vi "Test Register Path.vi"() -> ()   [LabVIEW 2021, in "Path Utilities.lvlib"]
doc: "Unit Test for \"Register Path.vi\"."
uses:
  Path Utilities.lvlib
panel:
  out "Cleared Paths":path[](array[path])
  out "Result":bool
  in  "Tests":T1(tab)
  out "Test 1":T2
  out "Test 2":T2
  out "Test 3":T2
  out "Test 4":T2
  out "Test 5":T2
  out "Test 6":T2
  out "Test 7":T2
  out "Test 8":T2
  out "Test 9":T2
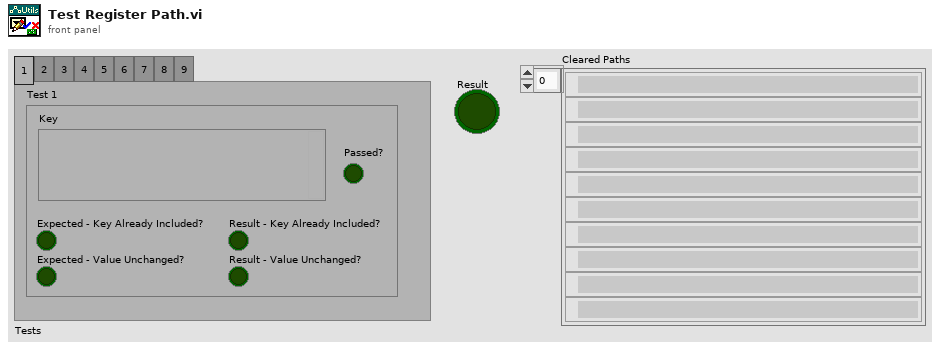
[diagram p1: front panel]
types:
  T1 = enum32{"1", "2", "3", "4", "5", "6", "7", "8", "9"}
  T2 = cluster{"Key":variant, "Result - Key Already Included?":bool, "Result - Value Unchanged?":bool, "Expected - Key Already Included?":bool, "Expected - Value Unchanged?":bool, "Passed?":bool}
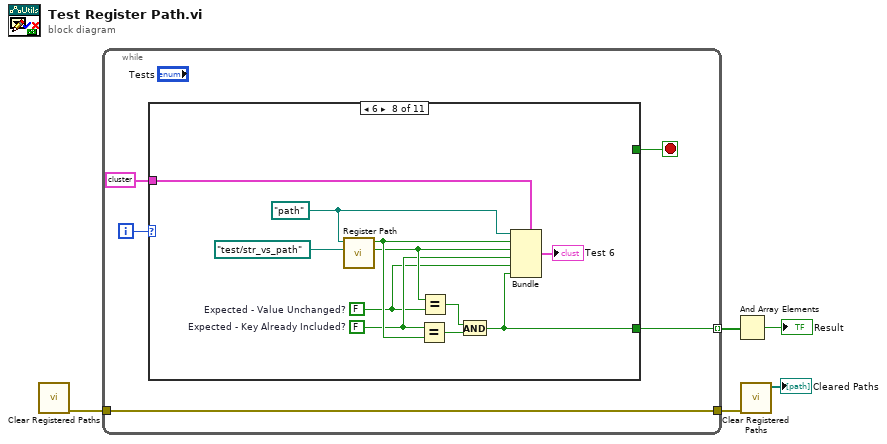
[diagram p0: block diagram]
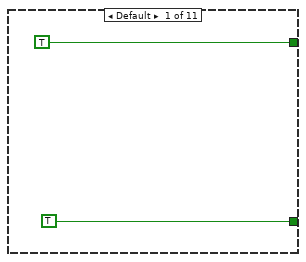
[diagram p2: hidden frame]
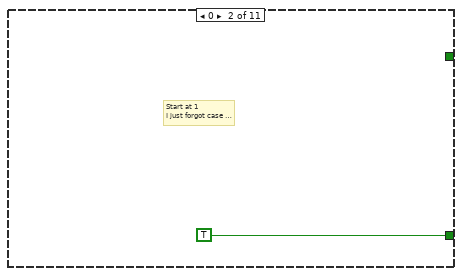
[diagram p3: hidden frame]
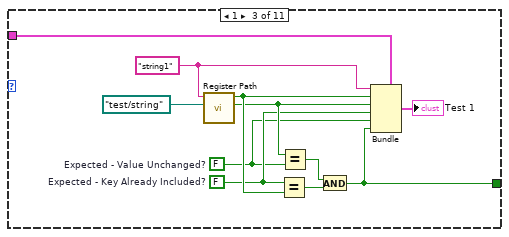
[diagram p4: hidden frame]
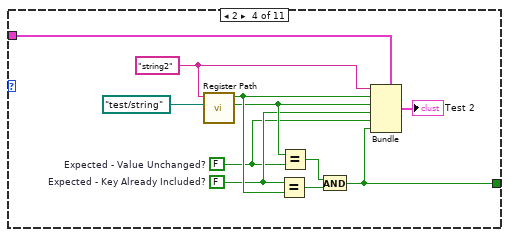
[diagram p5: hidden frame]
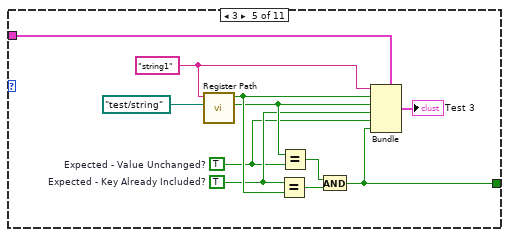
[diagram p6: hidden frame]
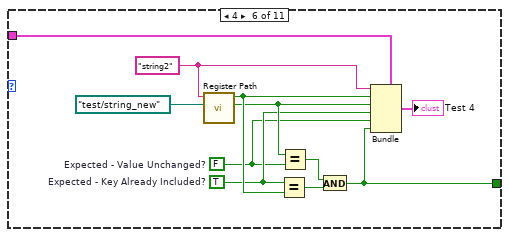
[diagram p7: hidden frame]
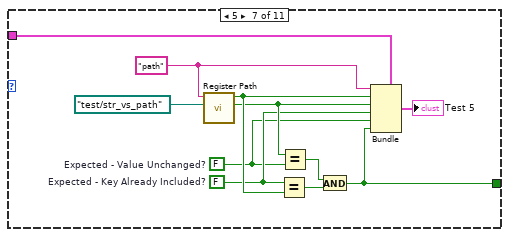
[diagram p8: hidden frame]
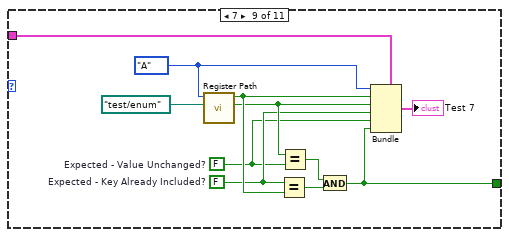
[diagram p9: hidden frame]
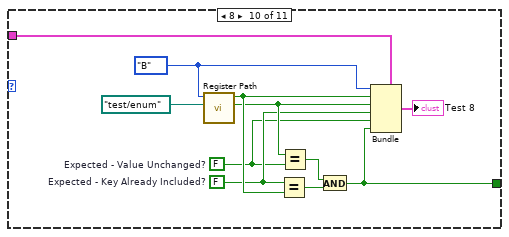
[diagram p10: hidden frame]
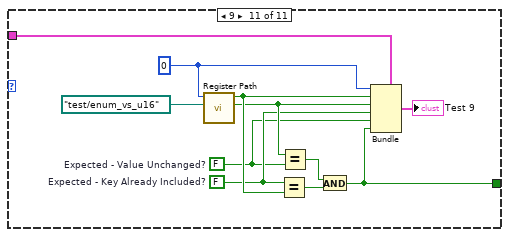
[diagram p11: hidden frame]
diagram:
  n1 = call "Clear Registered Paths.vi"() -> ("error out"=w3:errorcluster)  [unwired: 10 in, 1 out]
  n2 = while {
    tunnel: [w7] -> w5 mode=indexing
    tunnel: w3 -> [w6]
    tunnel: [w6] -> w2
    i -> [w10]
    stop <- w9 stop-if-true
    n3 = case shown="6" w10 {
      tunnel: [TRUE _ _ _ _ _ _ _ _ _ _] -> w9
      tunnel: T2 {"Key"=variant, "Result - Key Already Included?"=FALSE, "Result - Value Unchanged?"=FALSE, "Expected - Key Already Included?"=FALSE, "Expected - Value Unchanged?"=FALSE, "Passed?"=FALSE} ("Test 1") -> [_ _ w22 w33 w44 w55 w66 w77 w88 w99 w110]
      tunnel: [TRUE TRUE w14 w25 w36 w47 w58 w69 w80 w91 w103] -> w7
      frame Default {
      }
      frame 0 {
        # "Start at 1\nI just forgot case 0 lol"
      }
      frame 1 {
        w15 = FALSE  # Expected - Value Unchanged?
        w16 = FALSE  # Expected - Key Already Included?
        w21 = "string1"
        n4 = call "Register Path.vi"("Path"=path "test/string", "Key"=w21) -> ("Value Unchanged?"=w17:bool, "Key Already Included?"=w20:bool)  [unwired: 7 in, 1 out]
        n5 = Equal?(x=w16, y=w20) -> (x = y?=w19:bool)
        n6 = Equal?(x=w17, y=w15) -> (x = y?=w18:bool)
        n7 = And(x=w18, y=w19) -> (x .and. y?=w14:bool)
        n8 = Bundle(cluster=w22, "Key"=w21, "Result - Key Already Included?"=w20, "Result - Value Unchanged?"=w17, "Expected - Key Already Included?"=w16, "Expected - Value Unchanged?"=w15, "Passed?"=w14) -> (→"Test 1":T2)
      }
      frame 2 {
        w26 = FALSE  # Expected - Value Unchanged?
        w27 = FALSE  # Expected - Key Already Included?
        w32 = "string2"
        n9 = call "Register Path.vi"("Path"=path "test/string", "Key"=w32) -> ("Value Unchanged?"=w28:bool, "Key Already Included?"=w31:bool)  [unwired: 7 in, 1 out]
        n10 = Equal?(x=w27, y=w31) -> (x = y?=w30:bool)
        n11 = Equal?(x=w28, y=w26) -> (x = y?=w29:bool)
        n12 = And(x=w29, y=w30) -> (x .and. y?=w25:bool)
        n13 = Bundle(cluster=w33, "Key"=w32, "Result - Key Already Included?"=w31, "Result - Value Unchanged?"=w28, "Expected - Key Already Included?"=w27, "Expected - Value Unchanged?"=w26, "Passed?"=w25) -> (→"Test 2":T2)
      }
      frame 3 {
        w37 = TRUE  # Expected - Value Unchanged?
        w38 = TRUE  # Expected - Key Already Included?
        w43 = "string1"
        n14 = call "Register Path.vi"("Path"=path "test/string", "Key"=w43) -> ("Value Unchanged?"=w39:bool, "Key Already Included?"=w42:bool)  [unwired: 7 in, 1 out]
        n15 = Equal?(x=w38, y=w42) -> (x = y?=w41:bool)
        n16 = Equal?(x=w39, y=w37) -> (x = y?=w40:bool)
        n17 = And(x=w40, y=w41) -> (x .and. y?=w36:bool)
        n18 = Bundle(cluster=w44, "Key"=w43, "Result - Key Already Included?"=w42, "Result - Value Unchanged?"=w39, "Expected - Key Already Included?"=w38, "Expected - Value Unchanged?"=w37, "Passed?"=w36) -> (→"Test 3":T2)
      }
      frame 4 {
        w48 = FALSE  # Expected - Value Unchanged?
        w49 = TRUE  # Expected - Key Already Included?
        w54 = "string2"
        n19 = call "Register Path.vi"("Path"=path "test/string_new", "Key"=w54) -> ("Value Unchanged?"=w50:bool, "Key Already Included?"=w53:bool)  [unwired: 7 in, 1 out]
        n20 = Equal?(x=w49, y=w53) -> (x = y?=w52:bool)
        n21 = Equal?(x=w50, y=w48) -> (x = y?=w51:bool)
        n22 = And(x=w51, y=w52) -> (x .and. y?=w47:bool)
        n23 = Bundle(cluster=w55, "Key"=w54, "Result - Key Already Included?"=w53, "Result - Value Unchanged?"=w50, "Expected - Key Already Included?"=w49, "Expected - Value Unchanged?"=w48, "Passed?"=w47) -> (→"Test 4":T2)
      }
      frame 5 {
        w59 = FALSE  # Expected - Value Unchanged?
        w60 = FALSE  # Expected - Key Already Included?
        w65 = "path"
        n24 = call "Register Path.vi"("Path"=path "test/str_vs_path", "Key"=w65) -> ("Value Unchanged?"=w61:bool, "Key Already Included?"=w64:bool)  [unwired: 7 in, 1 out]
        n25 = Equal?(x=w60, y=w64) -> (x = y?=w63:bool)
        n26 = Equal?(x=w61, y=w59) -> (x = y?=w62:bool)
        n27 = And(x=w62, y=w63) -> (x .and. y?=w58:bool)
        n28 = Bundle(cluster=w66, "Key"=w65, "Result - Key Already Included?"=w64, "Result - Value Unchanged?"=w61, "Expected - Key Already Included?"=w60, "Expected - Value Unchanged?"=w59, "Passed?"=w58) -> (→"Test 5":T2)
      }
      frame 6 {
        w70 = path "path" ("Path")
        w71 = FALSE  # Expected - Value Unchanged?
        w72 = FALSE  # Expected - Key Already Included?
        n29 = call "Register Path.vi"("Path"=path "test/str_vs_path", "Key"=w70) -> ("Value Unchanged?"=w73:bool, "Key Already Included?"=w76:bool)  [unwired: 7 in, 1 out]
        n30 = Equal?(x=w72, y=w76) -> (x = y?=w75:bool)
        n31 = Equal?(x=w73, y=w71) -> (x = y?=w74:bool)
        n32 = And(x=w74, y=w75) -> (x .and. y?=w69:bool)
        n33 = Bundle(cluster=w77, "Key"=w70, "Result - Key Already Included?"=w76, "Result - Value Unchanged?"=w73, "Expected - Key Already Included?"=w72, "Expected - Value Unchanged?"=w71, "Passed?"=w69) -> (→"Test 6":T2)
      }
      frame 7 {
        w81 = enum16{"A", "B", "C"}."A"
        w82 = FALSE  # Expected - Value Unchanged?
        w83 = FALSE  # Expected - Key Already Included?
        n34 = call "Register Path.vi"("Path"=path "test/enum", "Key"=w81) -> ("Value Unchanged?"=w84:bool, "Key Already Included?"=w87:bool)  [unwired: 7 in, 1 out]
        n35 = Equal?(x=w83, y=w87) -> (x = y?=w86:bool)
        n36 = Equal?(x=w84, y=w82) -> (x = y?=w85:bool)
        n37 = And(x=w85, y=w86) -> (x .and. y?=w80:bool)
        n38 = Bundle(cluster=w88, "Key"=w81, "Result - Key Already Included?"=w87, "Result - Value Unchanged?"=w84, "Expected - Key Already Included?"=w83, "Expected - Value Unchanged?"=w82, "Passed?"=w80) -> (→"Test 7":T2)
      }
      frame 8 {
        w92 = enum16{"A", "B", "C"}."B"
        w93 = FALSE  # Expected - Value Unchanged?
        w94 = FALSE  # Expected - Key Already Included?
        n39 = call "Register Path.vi"("Path"=path "test/enum", "Key"=w92) -> ("Value Unchanged?"=w95:bool, "Key Already Included?"=w98:bool)  [unwired: 7 in, 1 out]
        n40 = Equal?(x=w94, y=w98) -> (x = y?=w97:bool)
        n41 = Equal?(x=w95, y=w93) -> (x = y?=w96:bool)
        n42 = And(x=w96, y=w97) -> (x .and. y?=w91:bool)
        n43 = Bundle(cluster=w99, "Key"=w92, "Result - Key Already Included?"=w98, "Result - Value Unchanged?"=w95, "Expected - Key Already Included?"=w94, "Expected - Value Unchanged?"=w93, "Passed?"=w91) -> (→"Test 8":T2)
      }
      frame 9 {
        w102 = u16 0
        w104 = FALSE  # Expected - Value Unchanged?
        w105 = FALSE  # Expected - Key Already Included?
        n44 = call "Register Path.vi"("Path"=path "test/enum_vs_u16", "Key"=w102) -> ("Value Unchanged?"=w106:bool, "Key Already Included?"=w109:bool)  [unwired: 7 in, 1 out]
        n45 = Equal?(x=w105, y=w109) -> (x = y?=w108:bool)
        n46 = Equal?(x=w106, y=w104) -> (x = y?=w107:bool)
        n47 = And(x=w107, y=w108) -> (x .and. y?=w103:bool)
        n48 = Bundle(cluster=w110, "Key"=w102, "Result - Key Already Included?"=w109, "Result - Value Unchanged?"=w106, "Expected - Key Already Included?"=w105, "Expected - Value Unchanged?"=w104, "Passed?"=w103) -> (→"Test 9":T2)
      }
    }
  }
  n49 = And Array Elements(Boolean array=w5) -> (logical AND=→"Result":bool)
  n50 = call "Clear Registered Paths.vi"("error in (no error)"=w2) -> ("Cleared Paths"=→"Cleared Paths":path[])  [unwired: 9 in, 1 out]
